vi "api_mqttConnect.vi"(0 "mqtt.lvclass in":refnum<class "mqtt.lvclass">, 11 "error in (no error)":errorcluster) -> (4 "mqtt.lvclass out":refnum<class "mqtt.lvclass">, 6 "success":bool, 8 "connStatus":T1=enum."Connection refused: not authorized", 10 "sessionPresent":bool, 15 "error out":errorcluster)   [LabVIEW 2018, in "labview-mqtt.lvlib" / "mqtt.lvclass"]
uses:
  mqtt.lvclass
  mqttTypedef/mqttConnectionStatus.ctl
  mqttCmd/mqttCmdConnect/mqttCmdConnect.lvclass
  D:/OneDrive/_WorkingOn/IECube/MQTT LabVIEW/mqtt-LabVIEW-master-yao/src/class/mqtt/mqttCmd/mqttCmd.lvclass
  mqttTypedef/mqttQOSlevel.ctl
  mqttTypedef/mqttMessageType.ctl
  mqttCmd/mqttCmdConnect/mqttCmdConnect.lvclass/mqttCmdConnect.ctl
  mqttCmd/mqttCmd.lvclass/mqttCmd.ctl
  mqttCmd/mqttCmd.lvclass
  labview-mqtt.lvlib
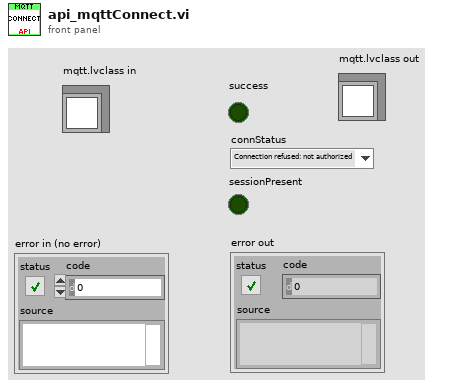
[diagram p1: front panel]
types:
  T1 = typedef "labview-mqtt.lvlib/mqttConnectionStatus.ctl" = enum16{"Connection accepted", "Connection refused: unacceptable protocol version", "Connection refused: identifier rejected", "Connection refused: Server unavailable", "Connection refused: bad user name or password", "Connection refused: not authorized"}
  T2 = typedef "labview-mqtt.lvlib/mqttMessageType.ctl" = enum32{"Reserved", "CONNECT", "CONNACK", "PUBLISH", "PUBACK", "PUBREC", "PUBREL", "PUBCOMP", "SUBSCRIBE", "SUBACK", "UNSUBSCRIBE", "UNSUBACK", "PINGREQ", "PINGRESP", "DISCONNECT", "Reserved2"}
  T3 = typedef "labview-mqtt.lvlib/mqttQOSlevel.ctl" = enum8{"At most once", "At least once", "Exactly once", "Reserved"}
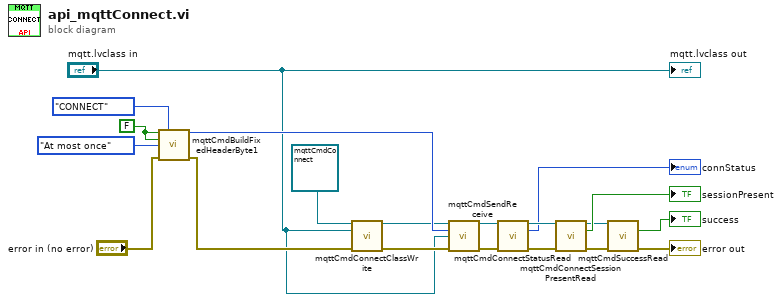
[diagram p0: block diagram]
diagram:
  w17 = FALSE
  n1 = call "mqttCmdBuildFixedHeaderByte1.vi"("retain(F)"=w17, "MessageType"=mqttMessageType."CONNECT", "duplicate(F)"=w17, "QoS (At most once)"=mqttQOSlevel."At most once", "error in (no error)"="error in (no error)") -> ("byte1"=w19:u8, "error out"=w15:errorcluster)  [unwired: 9 in]
  n2 = call "mqttCmdConnectClassWrite.vi"("mqttConnect in"=refnum<class "mqttCmdConnect.lvclass"> refnum ("mqttConnect.lvclass"), "mqtt.lvclass"="mqtt.lvclass in", "error in (no error)"=w15) -> ("mqttConnect out"=w13:refnum<class "mqttCmdConnect.lvclass">, "error out"=w12:errorcluster)  [unwired: 11 in]
  n3 = call "mqttCmdSendReceive.vi"("mqttConnect in"=w13, "byte1"=w19, "mqtt in"="mqtt.lvclass in", "error in (no error)"=w12) -> ("mqttConnect out"=w3:refnum<class "mqttCmdConnect.lvclass">, "error out"=w2:errorcluster)  [unwired: 9 in, 1 out]
  n4 = call "mqttCmdConnectStatusRead.vi"("mqttConnect in"=w3, "error in (no error)"=w2) -> ("mqttConnect out"=w10:refnum<class "mqttCmdConnect.lvclass">, "connStatus"=→"connStatus":T1, "error out"=w11:errorcluster)  [unwired: 11 in]
  n5 = call "mqttCmdConnectSessionPresentRead.vi"("mqttConnect in"=w10, "error in (no error)"=w11) -> ("mqttConnect out"=w5:refnum<class "mqttCmdConnect.lvclass">, "sessionPresent"=→"sessionPresent":bool, "error out"=w7:errorcluster)  [unwired: 11 in]
  n6 = call "mqttCmdSuccessRead.vi"("mqttBrokerCommand in"=w5, "error in (no error)"=w7) -> ("success"=→"success":bool, "error out"=→"error out":errorcluster)  [unwired: 11 in, 1 out]
  "mqtt.lvclass out" <- "mqtt.lvclass in"
